vi "security system.vi"() -> ()   [LabVIEW 2020]
uses:
  <vilib>/Instr/_visa.llb/VISA Configure Serial Port (Instr).vi
panel:
  out "path 2":path
  out "error out 2":errorcluster
  in  "file path (use dialog) 2":path
  in  "History":string[][](table)
  out "Sound":bool
  out "Temp alert":dbl(knob) scale=0.0..200.0
  out "Motion":bool
  out "Vibration":bool
  out "Temparature":dbl
  out "dist slide":u8(slide) scale=0.0..100.0
  in  "Off / On":bool
  in  "Select com port":refnum<visa-resource-name>
  out "dist (cm)":dbl
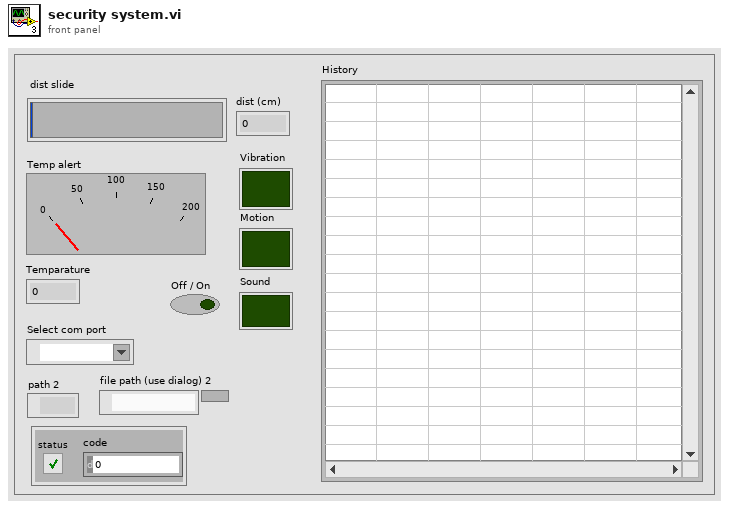
[diagram p1: front panel]
types:
  T1 = enum16{"open", "replace", "create", "open or create", "replace or create", "replace or create with confirmation"}
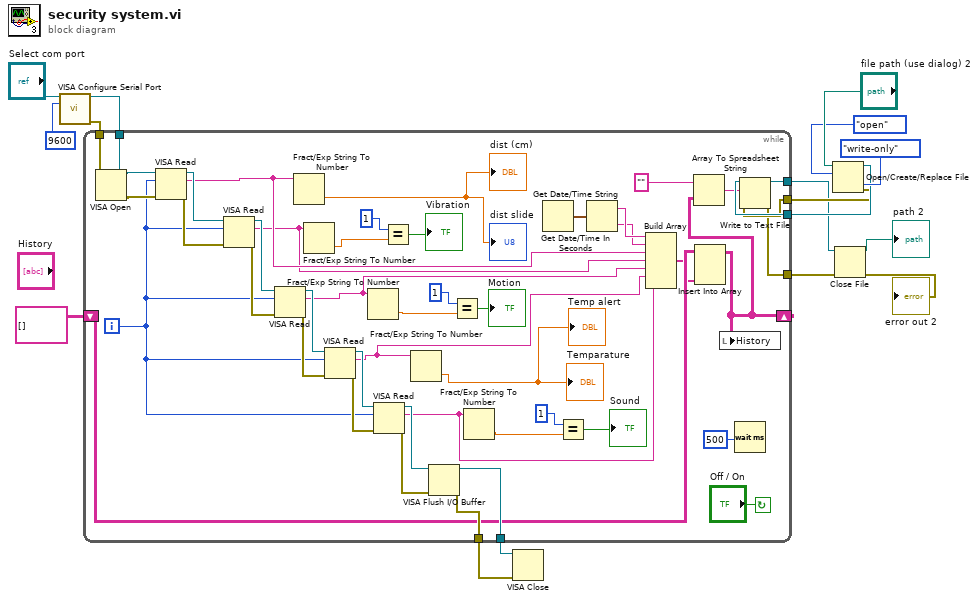
[diagram p0: block diagram]
diagram:
  n1 = call-poly "VISA Configure Serial Port"("VISA resource name"="Select com port", "baud rate (9600)"=u32 9600) -> ("VISA resource name out"=w14:refnum<visa-resource-name>, "error out"=w13:errorcluster)  [unwired: 12 in]
  n2 = Open/Create/Replace File(file path (use dialog)="file path (use dialog) 2", operation (0:open)=T1."open", access (0:read/write)=enum16{"read/write", "read-only", "write-only"}."write-only") -> (refnum out=w4:refnum<file>, error out=w3:errorcluster)  [unwired: 3 in, 1 out]
  n3 = while {
    tunnel: w14 -> [w61]
    tunnel: w13 -> [w60]
    tunnel: [w56] -> w12
    tunnel: [w55] -> w11
    shift-right: [w17] -> _
    shift-left: string[][] [] -> [w30]
    tunnel: w4 -> [w24]
    tunnel: w3 -> [w23]
    tunnel: [w22] -> w2
    tunnel: [w21] -> w1
    i -> [w48]
    stop <- "Off / On" continue-if-true
    n4 = VISA Open(error in (no error)=w60, VISA resource name=w61) -> (VISA resource name=w63:refnum<visa-resource-name>, error out=w62:errorcluster)  [unwired: 3 in]
    n5 = VISA Read(VISA resource name=w63, byte count=w48, error in (no error)=w62) -> (VISA resource name out=w58:refnum<visa-resource-name>, read buffer=w29:string, error out=w57:errorcluster)  [unwired: 1 out]
    n6 = VISA Read(VISA resource name=w58, byte count=w48, error in (no error)=w57) -> (VISA resource name out=w54:refnum<visa-resource-name>, read buffer=w28:string, error out=w53:errorcluster)  [unwired: 1 out]
    n7 = VISA Read(VISA resource name=w54, byte count=w48, error in (no error)=w53) -> (VISA resource name out=w52:refnum<visa-resource-name>, read buffer=w27:string, error out=w51:errorcluster)  [unwired: 1 out]
    n8 = Fract/Exp String To Number(string=w29) -> (number=→"dist (cm)" →"dist slide":dbl)  [unwired: 3 in, 1 out]
    n9 = Fract/Exp String To Number(string=w28) -> (number=w45:dbl)  [unwired: 3 in, 1 out]
    n10 = VISA Read(VISA resource name=w52, byte count=w48, error in (no error)=w51) -> (VISA resource name out=w50:refnum<visa-resource-name>, read buffer=w26:string, error out=w49:errorcluster)  [unwired: 1 out]
    n11 = Fract/Exp String To Number(string=w27) -> (number=w41:dbl)  [unwired: 3 in, 1 out]
    n12 = VISA Read(VISA resource name=w50, byte count=w48, error in (no error)=w49) -> (VISA resource name out=w47:refnum<visa-resource-name>, read buffer=w25:string, error out=w46:errorcluster)  [unwired: 1 out]
    n13 = Equal?(x=1, y=w45) -> (x = y?=→"Vibration":bool)
    n14 = Fract/Exp String To Number(string=w26) -> (number=→"Temparature" →"Temp alert":dbl)  [unwired: 3 in, 1 out]
    n15 = VISA Flush I/O Buffer(VISA resource name=w47, error in (no error)=w46) -> (VISA resource name out=w56:refnum<visa-resource-name>, error out=w55:errorcluster)  [unwired: 1 in]
    n16 = Equal?(x=1, y=w41) -> (x = y?=→"Motion":bool)
    n17 = Fract/Exp String To Number(string=w25) -> (number=w38:dbl)  [unwired: 3 in, 1 out]
    n18 = Get Date/Time In Seconds() -> (seconds since 1Jan1904=w33:timestamp)
    n19 = Equal?(x=1, y=w38) -> (x = y?=→"Sound":bool)
    n20 = Get Date/Time String(seconds (now)=w33) -> (date string=w32:string, time string=w31:string)  [unwired: 2 in]
    n21 = Build Array(w32, w31, w29, w28, w27, w26, w25) -> (w18:string[])
    n22 = Insert Into Array(array=w30, new element=w18) -> (w17:string[][])  [unwired: 2 in]
    n23 = Array To Spreadsheet String(array=w17, 3:"") -> (spreadsheet string=w20:string)  [unwired: 1 in]
    n24 = local write "History"(w17) -> ()
    n25 = Wait (ms)(milliseconds to wait=u32 500 ("baud rate (9600)")) -> ()  [unwired: 1 out]
    n26 = Write to Text File(file (use dialog)=w24, text=w20, error in=w23) -> (refnum out=w22:refnum<file>, error out=w21:errorcluster)  [unwired: 1 in, 1 out]
  }
  n27 = VISA Close(VISA resource name=w12, error in (no error)=w11) -> ()  [unwired: 1 out]
  n28 = Close File(refnum=w2, error in=w1) -> (path=→"path 2":path, error out=→"error out 2":errorcluster)
